vi "3DBaxter.vi"() -> ()   [LabVIEW 2012]
uses:
  <vilib>/Utility/miscctls.llb/LVRGBAColorTypeDef.ctl
  <vilib>/picture/3D Picture Control/NI_3D Picture Control.lvlib
panel:
  in  "Tab Control":enum32{"Body", "Left Arm"}(tab)=enum."Left Arm"
  in  "Cylinder":T1={"Height"=0.5, "Radius"=0.15, "Color Box"=2817871, "Alpha"=1.0, "Detail"=1.0}
  in  "Axis":cluster{"X":sgl, "Y":sgl, "Z":sgl}={"X"=1.0, "Y"=0.0, "Z"=0.0}
  in  "Translation":cluster{"X":sgl, "Y":sgl, "Z":sgl}={"X"=0.0, "Y"=0.5, "Z"=0.0}
  in  "Cube":T2={"X"=1.0, "Y"=1.0, "Z"=0.3, "Color Box"=10987431, "Alpha"=1.0}
  out "3D Picture 2":refnum<vi>(3d-picture)
  out "3D Picture":refnum<vi>(3d-picture)
  in  "Joint States":T3(array[cluster])=[{"Joint Name"="right_s0", "Position"=45.0, "Velocity"=0.0, "Effort"=0.0}, {"Joint Name"="right_s1", "Position"=45.0, "Velocity"=0.0, "Effort"=0.0}]
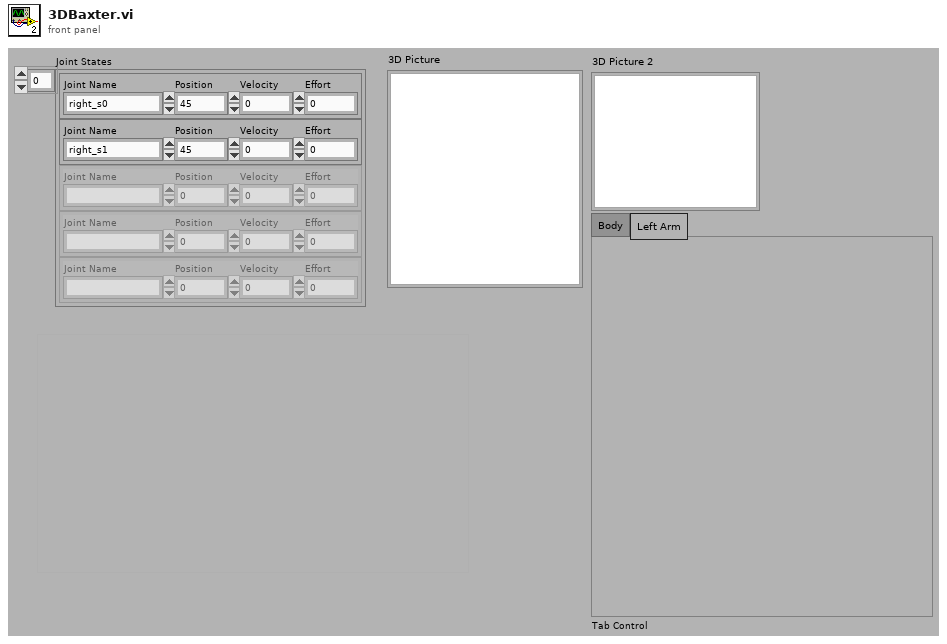
[diagram p1: front panel]
types:
  T1 = cluster{"Height":sgl, "Radius":sgl, "Color Box":u32, "Alpha":sgl, "Detail":sgl}
  T2 = cluster{"X":sgl, "Y":sgl, "Z":sgl, "Color Box":u32, "Alpha":sgl}
  T3 = cluster{"Joint Name":string, "Position":dbl, "Velocity":dbl, "Effort":dbl}[]
  T4 = typedef "LVRGBAColorTypeDef.ctl" = cluster{"Red":sgl, "Green":sgl, "Blue":sgl, "Alpha":sgl}
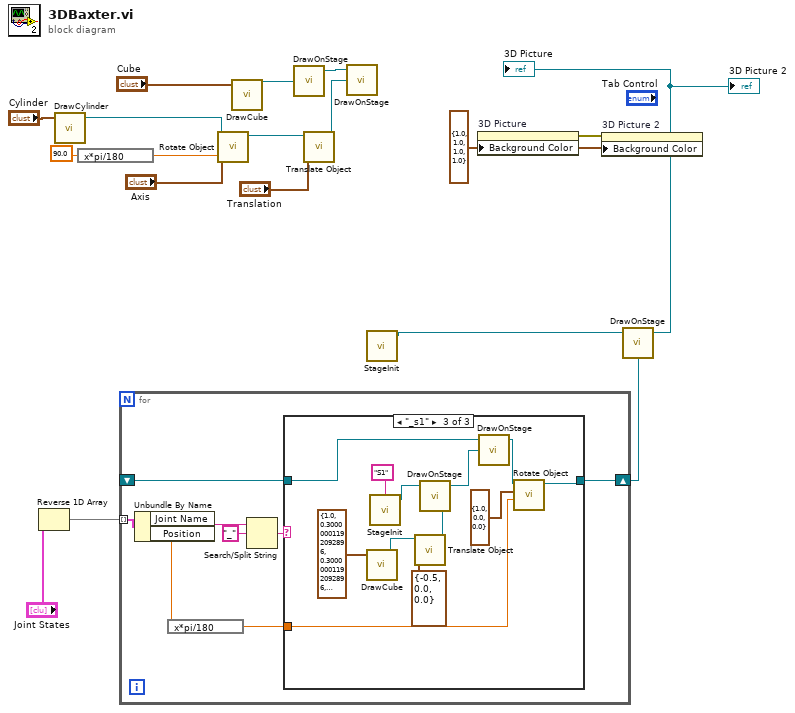
[diagram p0: block diagram]
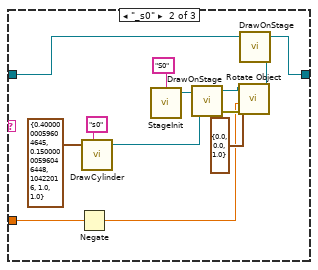
[diagram p3: hidden frame]
diagram:
  w6 = T4 {"Red"=1.0, "Green"=1.0, "Blue"=1.0, "Alpha"=1.0} ("Background Color")
  n1 = Reverse 1D Array(array="Joint States") -> (reversed array=w4:T3)
  n2 = call <userlib>:"DrawCylinder.vi"("Cylinder"="Cylinder") -> ("object out"=w12:refnum<vi>)  [unwired: 5 in, 1 out]
  n3 = expression code="x*pi/180"(sgl 90.0 ("Angle")) -> (w8:sgl)
  n4 = for {
    tunnel: w4 -> [w26] mode=indexing
    shift-right: [w24] -> w2
    shift-left: _ -> [w25]
    n5 = Unbundle By Name(w26) -> ("Joint Name"=w23:string, "Position"=w20:dbl)
    n6 = expression code="x*pi/180"(w20) -> (w19:dbl)
    n7 = Search/Split String(string=w23, search string/char (-)="_") -> (match + rest of string=w21:string)  [unwired: 1 in, 2 out]
    n8 = case shown="\"_s1\"" w21 {
      tunnel: w25 -> [w27 w30 w43]
      tunnel: [w27 w28 w41] -> w24
      tunnel: w19 -> [_ w36 w50]
      frame Default {
      }
      frame "_s0" {
        n9 = Negate(x=w36) -> (-x=w34:dbl)
        n10 = call <userlib>:"DrawCylinder.vi"("Cylinder"=T1 {"Height"=0.4, "Radius"=0.15, "Color Box"=10422016, "Alpha"=1.0, "Detail"=1.0} ("shoulder 0"), "Name"="s0") -> ("object out"=w38:refnum<vi>)  [unwired: 4 in, 1 out]
        n11 = call <userlib>:"StageInit.vi"("Name"="S0") -> ("Stage out"=w32:refnum<vi>)  [unwired: 3 in, 1 out]
        n12 = call <userlib>:"DrawOnStage.vi"("object in"=w38, "Stage in"=w32) -> ("error out"=w37:errorcluster, "Stage out"=w31:refnum<vi>)  [unwired: 1 in, 1 out]
        n13 = call <vilib>:"Rotate Object.vi"("error in (no error)"=w37, "Angle"=w34, "Axis"=cluster{"X":sgl, "Y":sgl, "Z":sgl} {"X"=0.0, "Y"=0.0, "Z"=1.0}, "Scene.Object In"=w31) -> ("Scene.Object Out"=w29:refnum<vi>)  [unwired: 6 in, 1 out]
        n14 = call <userlib>:"DrawOnStage.vi"("object in"=w29, "Stage in"=w30) -> ("Stage out"=w28:refnum<vi>)  [unwired: 1 in, 2 out]
      }
      frame "_s1" {
        n15 = call <userlib>:"DrawCube.vi"("Cube"=T2 {"X"=1.0, "Y"=0.3, "Z"=0.3, "Color Box"=15666944, "Alpha"=1.0} ("Upper Arm")) -> ("object out"=w48:refnum<vi>)  [unwired: 5 in, 1 out]
        n16 = call <userlib>:"StageInit.vi"("Name"="S1") -> ("Stage out"=w46:refnum<vi>)  [unwired: 3 in, 1 out]
        n17 = call <vilib>:"Translate Object.vi"("Translation"=cluster{"X":sgl, "Y":sgl, "Z":sgl} {"X"=-0.5, "Y"=0.0, "Z"=0.0}, "Scene.Object In"=w48) -> ("Scene.Object Out"=w47:refnum<vi>)  [unwired: 8 in, 1 out]
        n18 = call <userlib>:"DrawOnStage.vi"("object in"=w47, "Stage in"=w46) -> ("Stage out"=w44:refnum<vi>)  [unwired: 1 in, 2 out]
        n19 = call <userlib>:"DrawOnStage.vi"("object in"=w44, "Stage in"=w43) -> ("Stage out"=w42:refnum<vi>)  [unwired: 1 in, 2 out]
        n20 = call <vilib>:"Rotate Object.vi"("Angle"=w50, "Axis"=cluster{"X":sgl, "Y":sgl, "Z":sgl} {"X"=1.0, "Y"=0.0, "Z"=0.0}, "Scene.Object In"=w42) -> ("Scene.Object Out"=w41:refnum<vi>)  [unwired: 7 in, 1 out]
      }
    }
  }
  n21 = call <vilib>:"Rotate Object.vi"("Angle"=w8, "Axis"="Axis", "Scene.Object In"=w12) -> ("Scene.Object Out"=w11:refnum<vi>)  [unwired: 7 in, 1 out]
  n22 = call <userlib>:"DrawCube.vi"("Cube"="Cube") -> ("object out"=w13:refnum<vi>)  [unwired: 5 in, 1 out]
  n23 = call <userlib>:"DrawOnStage.vi"("object in"=w13) -> ("Stage out"=w15:refnum<vi>)  [unwired: 2 in, 2 out]
  n24 = call <vilib>:"Translate Object.vi"("Translation"="Translation", "Scene.Object In"=w11) -> ("Scene.Object Out"=w14:refnum<vi>)  [unwired: 8 in, 1 out]
  n25 = call <userlib>:"DrawOnStage.vi"("object in"=w14, "Stage in"=w15) -> ()  [unwired: 1 in, 3 out]
  n26 = call <userlib>:"StageInit.vi"() -> ("Stage out"=w3:refnum<vi>)  [unwired: 4 in, 1 out]
  n27 = property on="3D Picture" class="SceneGraphDisp (strict)"("Background Color"=w6) -> (error out=w7:errorcluster)  [unwired: 2 in, 1 out]
  n28 = property on="3D Picture 2" class="SceneGraphDisp (strict)"(error in=w7, "Background Color"=w6) -> ()  [unwired: 1 in, 2 out]
  n29 = call <userlib>:"DrawOnStage.vi"("object in"=w2, "Stage in"=w3) -> ("Stage out"=→"3D Picture" →"3D Picture 2":refnum<vi>)  [unwired: 1 in, 2 out]
